vi "1D Array Image Index.vi"(8 "error in (no error)":errorcluster, 10 "# Image":u32, 11 "Series Graph in":refnum<class "Series Graph.lvclass">) -> (0 "error out":errorcluster, 1 "Image Length":u32, 2 "Image Index":u32, 3 "Series Graph out":refnum<class "Series Graph.lvclass">)   [LabVIEW 2023, in "Series Graph.lvclass"]
uses:
  Series Graph.lvclass
  Series Graph.lvclass/Series Graph.ctl
  Base Graph/Base Graph.lvclass
  D:/git/Graph-Classes/graph-classes/Detail Graph/Detail Graph.lvclass
  D:/git/Graph-Classes/graph-classes/Base Graph/Base Graph.lvclass
  D:/git/Graph-Classes/graph-classes/Series Graph/Series Graph.lvclass
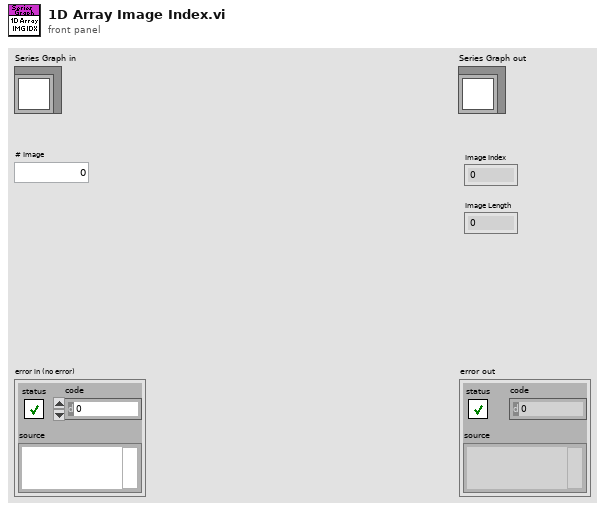
[diagram p1: front panel]
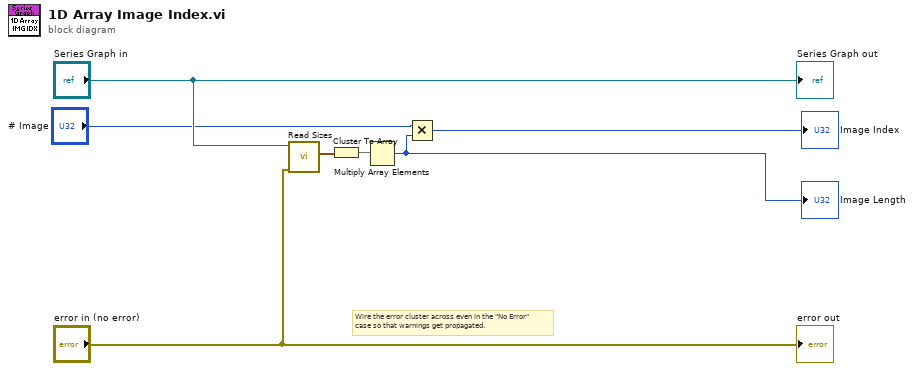
[diagram p0: block diagram]
diagram:
  # "Wire the error cluster across even in the \"No Error\"\ncase so that warnings get propagated."
  n1 = call "Read Sizes.vi"("error in (no error)"="error in (no error)", "TG Base Graph in"="Series Graph in") -> ("Sizes"=w1:cluster{"Height":u32, "Width":u32})  [unwired: 7 in, 2 out]
  n2 = Cluster To Array(cluster=w1) -> (array=w2:u32[])
  n3 = Multiply Array Elements(1:w2) -> (0:w3:u32)
  "Image Length" <- w3
  n4 = Multiply(x="# Image", y=w3) -> (x*y=→"Image Index":u32)
  "error out" <- "error in (no error)"
  "Series Graph out" <- "Series Graph in"
